vi "test_Task cRIO PWM in-out.vi"(8 "Error In":errorcluster) -> (0 "Error Out":errorcluster)   [LabVIEW 2023]
uses:
  Task/Task Base/Task Base.lvclass
  FGen/Virtual FGens/Virt Voltage Generator/Virt Voltage Generator.lvclass
  DIO/DO DAQmx Fixed Freq PWM CFG/DO DAQmx Fixed Freq PWM CFG.lvclass
  Sample Tasks/Sample Temp PWM Control/Sample Temp PWM Control.lvclass
  Devices/NEO480HTA/Real All CFG/Read All CFG.lvclass
  Task/Task Base/Task Base.lvclass/Task Base.ctl
  <vilib>/Utility/error.llb/Error Cluster From Error Code.vi
  Measure and Stimulus Subsystems/Measure and Stimulus Subsystems.lvclass
panel:
  in  "stop":bool
  in  "Temp Setpoint":dbl=23.0 format="%#_g °C"
  out "Waveform Chart Lossy":dbl(graph)
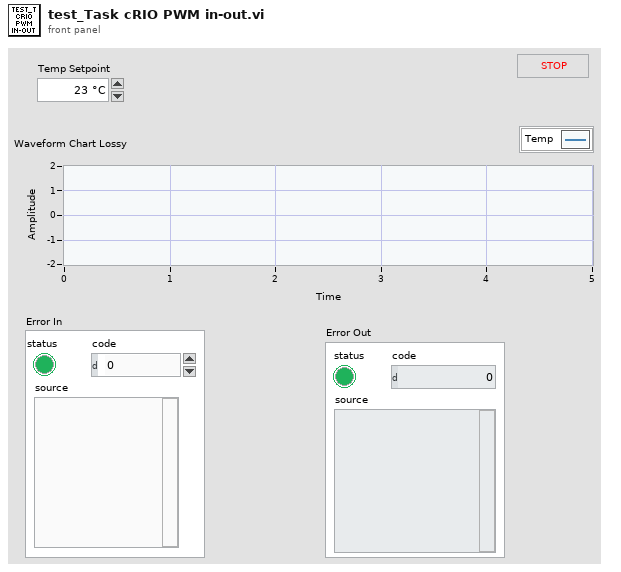
[diagram p1: front panel]
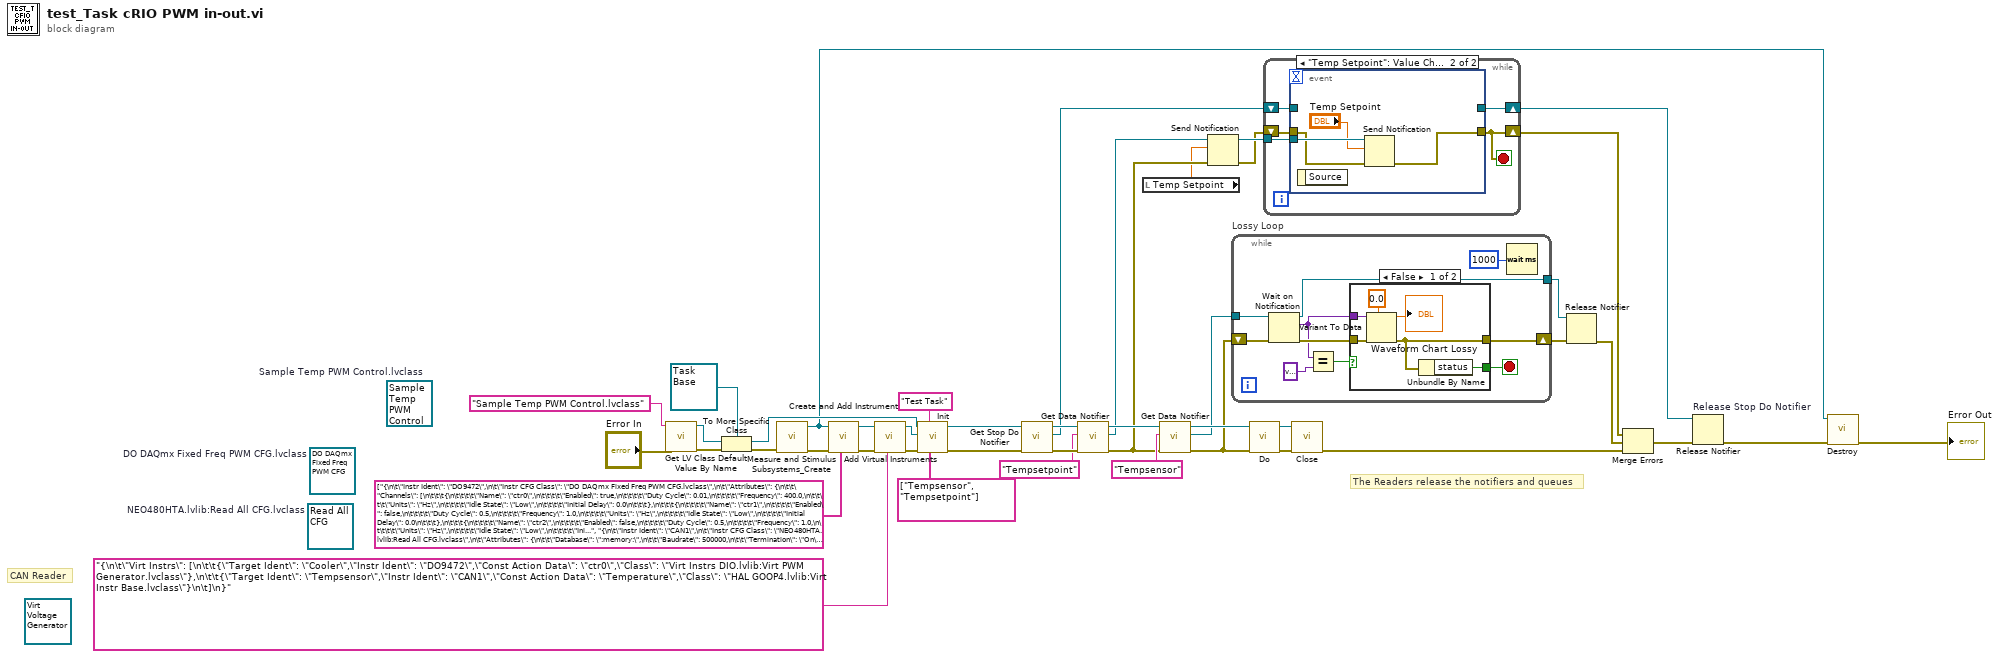
[diagram p0: block diagram]
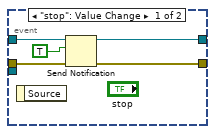
[diagram p3: hidden frame]
diagram:
  (unwired) refnum<class "Read All CFG.lvclass"> refnum  # NEO480HTA.lvlib:Read All CFG.lvclass
  (unwired) refnum<class "Sample Temp PWM Control.lvclass"> refnum  # Sample Temp PWM Control.lvclass
  (unwired) refnum<class "DO DAQmx Fixed Freq PWM CFG.lvclass"> refnum  # DO DAQmx Fixed Freq PWM CFG.lvclass
  (unwired) refnum<class "Virt Voltage Generator.lvclass"> refnum ("Virt Instrs FGen.lvlib:Virt Voltage Generator.lvclass")
  # "CAN Reader"
  # "The Readers release the notifiers and queues"
  n1 = call <vilib>:"Get LV Class Default Value By Name.vi"("error in (no error)"="Error In", "class name"="Sample Temp PWM Control.lvclass") -> ("error out"=w42:errorcluster, "object"=w39:refnum<class>)  [unwired: 8 in]
  n2 = To More Specific Class(target class=refnum<class "Task Base.lvclass"> refnum ("HAL GOOP4.lvlib:Task Base.lvclass"), reference=w39, error in=w42) -> (specific class reference=w35:refnum<class "Task Base.lvclass">, error out=w40:errorcluster)
  n3 = call "Measure and Stimulus Subsystems_Create.vi"("Error In"=w40) -> ("Error Out"=w44:errorcluster, "reference out"=w9:refnum<class "Measure and Stimulus Subsystems.lvclass">)  [unwired: 9 in]
  n4 = call "Create and Add Instrument.vi"("Physical Intr Configs"=string[] ["{\n\t\"Instr Ident\": \"DO9472\",\n\t\"Instr CFG Class\": \"DO DAQmx Fixed Freq PWM CFG.lvclass\",\n\t\"Attributes\": {\n\t\t\"Channels\": [\n\t\t\t{\n\t\t\t\t\"Name\": \"ctr0\",\n\t\t\t\t\"Enabled\": true,\n\t\t\t\t\"Duty Cycle\": 0.01,\n\t\t\t\t\"Frequency\": 400.0,\n\t\t\t\t\"Units\": \"Hz\",\n\t\t\t\t\"Idle State\": \"Low\",\n\t\t\t\t\"Initial Delay\": 0.0\n\t\t\t},\n\t\t\t{\n\t\t\t\t\"Name\": \"ctr1\",\n\t\t\t\t\"Enabled\": false,\n\t\t\t\t\"Duty Cycle\": 0.5,\n\t\t\t\t\"Frequency\": 1.0,\n\t\t\t\t\"Units\": \"Hz\",\n\t\t\t\t\"Idle State\": \"Low\",\n\t\t\t\t\"Initial Delay\": 0.0\n\t\t\t},\n\t\t\t{\n\t\t\t\t\"Name\": \"ctr2\",\n\t\t\t\t\"Enabled\": false,\n\t\t\t\t\"Duty Cycle\": 0.5,\n\t\t\t\t\"Frequency\": 1.0,\n\t\t\t\t\"Units\": \"Hz\",\n\t\t\t\t\"Idle State\": \"Low\",\n\t\t\t\t\"Initial Delay\": 0.0\n\t\t\t},\n\t\t\t{\n\t\t\t\t\"Name\": \"ctr3\",\n\t\t\t\t\"Enabled\": false,\n\t\t\t\t\"Duty Cycle\": 0.5,\n\t\t\t\t\"Frequency\": 1.0,\n\t\t\t\t\"Units\": \"Hz\",\n\t\t\t\t\"Idle State\": \"Low\",\n\t\t\t\t\"Initial Delay\": 0.0\n\t\t\t}\n\t\t],\n\t\t\"Timing\": {\n\t\t\t\"Samples per Channel\": 1000,\n\t\t\t\"Sample Mode\": \"Continuous Samples\",\n\t\t\t\"Sample Rate\": 0.0,\n\t\t\t\"Sample Clock Source\": \"Implicit\",\n\t\t\t\"Active Edge\": \"Rising\"\n\t\t},\n\t\t\"Trigger\": {\n\t\t\t\"Trigger Type\": \"No Trigger\"\n\t\t}\n\t}\n}", "{\n\t\"Instr Ident\": \"CAN1\",\n\t\"Instr CFG Class\": \"NEO480HTA.lvlib:Read All CFG.lvclass\",\n\t\"Attributes\": {\n\t\t\"Database\": \":memory:\",\n\t\t\"Baudrate\": 500000,\n\t\t\"Termination\": \"On\",\n\t\t\"CAN Frames\": [\n\t\t\t{\n\t\t\t\t\"Frame name\": \"Dew Point\",\n\t\t\t\t\"Identifier\": 1152,\n\t\t\t\t\"Extended Identifier\": false,\n\t\t\t\t\"Payload Length\":8,\n\t\t\t\t\"Timing Type\":\"Event Data\",\n\t\t\t\t\"Transmit Time\":0,\n\t\t\t\t\"Comment\":\"\"\n\t\t\t},\n\t\t\t{\n\t\t\t\t\"Frame name\": \"Dew Point Raw\",\n\t\t\t\t\"Identifier\": 1153,\n\t\t\t\t\"Extended Identifier\": false,\n\t\t\t\t\"Payload Length\":8,\n\t\t\t\t\"Timing Type\":\"Event Data\",\n\t\t\t\t\"Transmit Time\":0,\n\t\t\t\t\"Comment\":\"\"\n\t\t\t}\n\t\t],\n\t\t\"Acquire\": {\n\t\t\t\"Type\": \"Read Frame\"\n\t\t}\n\t}\n}"], "Error In"=w44, "reference in"=w9) -> ("Error Out"=w37:errorcluster, "reference out"=w36:refnum<class "Measure and Stimulus Subsystems.lvclass">)  [unwired: 7 in]
  n5 = call "Add Virtual Instruments.vi"("<JSON CFG>"="{\n\t\"Virt Instrs\": [\n\t\t{\"Target Ident\": \"Cooler\",\"Instr Ident\": \"DO9472\",\"Const Action Data\": \"ctr0\",\"Class\": \"Virt Instrs DIO.lvlib:Virt PWM Generator.lvclass\"},\n\t\t{\"Target Ident\": \"Tempsensor\",\"Instr Ident\": \"CAN1\",\"Const Action Data\": \"Temperature\",\"Class\": \"HAL GOOP4.lvlib:Virt Instr Base.lvclass\"}\n\t]\n}", "Error In"=w37, "reference in"=w36) -> ("Error Out"=w28:errorcluster, "reference out"=w34:refnum<class "Measure and Stimulus Subsystems.lvclass">)  [unwired: 7 in]
  n6 = call-dynamic "Init.vi"("Data Notifier Names"=string[] ["Tempsensor", "Tempsetpoint"], "Name"="Test Task", "error in (no error)"=w28, "MSS"=w34, "Task Base in"=w35) -> ("error out"=w20:errorcluster, "Task Base out"=w17:refnum<class "Task Base.lvclass">)  [unwired: 5 in]
  n7 = call "Get Stop Do Notifier.vi"("error in (no error)"=w20, "Task Base in"=w17) -> ("error out"=w19:errorcluster, "Stop Do"=w16:refnum<notifier>, "Task Base out"=w18:refnum<class "Task Base.lvclass">)  [unwired: 7 in]
  n8 = call "Get Data Notifier.vi"("error in (no error)"=w19, "Target Name"="Tempsetpoint" ("Name"), "Task Base in"=w18) -> ("error out"=w2:errorcluster, "Data Notifier"=w5:refnum<notifier>, "Task Base out"=w15:refnum<class "Task Base.lvclass">)  [unwired: 6 in]
  n9 = local read "Temp Setpoint"() -> (w1:dbl)
  n10 = call "Get Data Notifier.vi"("error in (no error)"=w2, "Target Name"="Tempsensor", "Task Base in"=w15) -> ("error out"=w6:errorcluster, "Data Notifier"=w11:refnum<notifier>, "Task Base out"=w14:refnum<class "Task Base.lvclass">)  [unwired: 6 in]
  n11 = Send Notification(notification=w1, notifier=w5, error in (no error)=w2) -> (notifier out=w4:refnum<notifier>, error out=w3:errorcluster)
  n12 = while "Lossy Loop" {
    tunnel: w11 -> [w50]
    shift-right: [w51] -> w27
    shift-left: w6 -> [w52]
    tunnel: [w49] -> w26
    stop <- w48 stop-if-true
    n13 = Wait on Notification(notifier=w50, error in (no error)=w52) -> (notifier out=w49:refnum<notifier>, notification=w46:variant, error out=w54:errorcluster)  [unwired: 2 in, 1 out]
    n14 = Equal?(x=w46, y=variant) -> (x = y?=w45:bool)
    n15 = case shown="False" w45 {
      selector: w45 -> [_ w62]
      tunnel: w54 -> [w60 w61]
      tunnel: [w58 w61] -> w51
      tunnel: [w55 w62] -> w48
      tunnel: w46 -> [w56 _]
      frame False {
        n16 = Variant To Data(error in=w60, type=0.0 ("Waveform"), Variant=w56) -> (data=→"Waveform Chart Lossy":dbl, error out=w58:errorcluster)
        n17 = Unbundle By Name(w58) -> ("status"=w55:bool)
      }
      frame True {
      }
    }
    n18 = Wait (ms)(milliseconds to wait=u32 1000) -> ()  [unwired: 1 out]
  }
  n19 = call-dynamic "Do.vi"("error in (no error)"=w6, "Task Base in"=w14) -> ("error out"=w31:errorcluster, "Task Base out"=w30:refnum<class "Task Base.lvclass">)  [unwired: 7 in, 1 out]
  n20 = while {
    tunnel: w4 -> [w65]
    shift-right: [w67] -> w21
    shift-left: w16 -> [w66]
    shift-right: [w64] -> w24
    shift-left: w3 -> [w63]
    stop <- w64 stop-if-true
    n21 = event shown="[1] \"Temp Setpoint\": Value Change" {
      selector: _ -> [_ _]
      dyn-events: _ -> [_ _]
      timeout: _ -> [_ _]
      tunnel: w66 -> [w72 _]
      tunnel: [w70 _] -> w67
      tunnel: [w69 w74] -> w64
      tunnel: w65 -> [_ w76]
      tunnel: w63 -> [w68 w73]
      event "stop": Value Change {
        n22 = event-data() -> ()  [unwired: 1 in, 1 out]
        n23 = Send Notification(notification=TRUE, notifier=w72, error in (no error)=w68) -> (notifier out=w70:refnum<notifier>, error out=w69:errorcluster)
      }
      event "Temp Setpoint": Value Change {
        n24 = event-data() -> ()  [unwired: 1 in, 1 out]
        n25 = Send Notification(notification="Temp Setpoint", notifier=w76, error in (no error)=w73) -> (error out=w74:errorcluster)  [unwired: 1 out]
      }
    }
  }
  n26 = call-dynamic "Close.vi"("error in (no error)"=w31, "Task Base in"=w30) -> ("error out"=w29:errorcluster)  [unwired: 8 in, 1 out]
  n27 = Release Notifier(notifier=w26, error in (no error)=w27) -> (error out=w23:errorcluster)  [unwired: 1 in, 2 out]
  n28 = Merge Errors(w24, w23, w29) -> (w25:errorcluster)
  n29 = Release Notifier "Release Stop Do Notifier"(notifier=w21, error in (no error)=w25) -> (error out=w22:errorcluster)  [unwired: 1 in, 2 out]
  n30 = call "Destroy.vi"("Error In"=w22, "reference in"=w9) -> ("Error Out"=→"Error Out":errorcluster)  [unwired: 8 in, 1 out]
